vi "dg645-full-controll2_legacy.vi"(0 "Cluster":T1={"ch AB delay(ns)"=0.0, "ch AB width(ns)"=1020.0, "ch CD delay(ns) "=0.0, "ch CD width(ns) "=2000.0, "ch EF delay(ns) "=0.0, "ch EF width(ns) "=1000.0, "ch GH delay(ns) "=0.0, "ch GH width(ns) "=1000.0} {"ch GH width(ns)" format="%^#_6e"; "ch GH delay(ns)" format="%^#_6e"; "ch EF width(ns)" format="%^#_6e"; "ch EF delay(ns)" format="%^#_6e"; "ch CD width(ns)" format="%^#_6e"; "ch CD delay(ns)" format="%^#_6e"; "ch AB width(ns)" format="%^#_6e"; "ch AB delay(ns)" format="%^#_6e"}) -> ()   [LabVIEW 2018]
doc: "This VI is an example of how to use the DG535 subVIs programmatically .\nThe DG535 TRIGGER.VI sets the trigger mode , internal/burst trigger rate , burst count , burst period , external threshold voltage , external trigger slope and impedance of the DG535 .\nErrors are reported if the trigger rate is too high or if the burst period is out-of-range .\nThe DG535 DELAY.VI sets the delay time of channel i to t seconds relative to channel j . A \"Delay Linkage Error\" is caused by an attempt to totally disconnect a time reference from T0 . A \"Delay Range Error\" is reported when the total time delay for a channel exceeds 999.999999999995 seconds .\nDG535 SET OUTPUT.VI sets the mode , load , output polarity, amplitude and offset of the OUTPUT BNC selected while the DG535 READ OUTPUT.VI reads and displays these values ."
panel:
  in  "Tab Control":enum32{"delay ", "output level"}(tab)
  in  "Inhibit trigger?":bool
  out "chH delay from G":string="8,+0.000000000000\r\n"
  out "chF delay from E":string="6,+0.000100000000\r\n"
  out "chG delay from T0":string="0,+0.000000000000\r\n"
  out "chE delay from T0":string="0,+0.000000000000\r\n"
  out "chC delay from T0":string="0,+0.000000000000\r\n"
  out "chD delay from C":string="4,+0.000001000000\r\n"
  out "chB delay from A":string="2,+0.000000370000\r\n"
  out "chA delay from T0":string
  in  "save?":bool
  in  "ch GH width(ns)":dbl=1000.0 format="%^#_6e"
  in  "ch GH delay(ns)":dbl format="%^#_6e"
  in  "ch EF width(ns)":dbl=1000.0 format="%^#_6e"
  in  "ch EF delay(ns)":dbl format="%^#_6e"
  in  "ch CD width(ns)":dbl=2000.0 format="%^#_6e"
  in  "ch CD delay(ns)":dbl format="%^#_6e"
  in  "ch AB width(ns)":dbl=1020.0 format="%^#_6e"
  in  "ch AB delay(ns)":dbl format="%^#_6e"
  in  "GPIB Address":string="15"
  out "error out":errorcluster
  in  "error in":errorcluster
  # "ps"
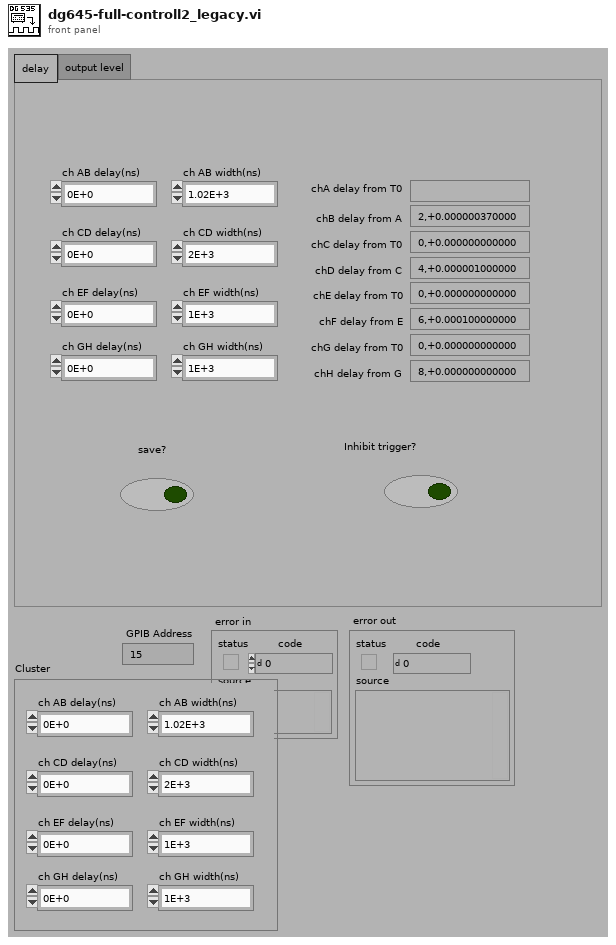
[diagram p1: front panel]
types:
  T1 = cluster{"ch AB delay(ns)":dbl, "ch AB width(ns)":dbl, "ch CD delay(ns) ":dbl, "ch CD width(ns) ":dbl, "ch EF delay(ns) ":dbl, "ch EF width(ns) ":dbl, "ch GH delay(ns) ":dbl, "ch GH width(ns) ":dbl}
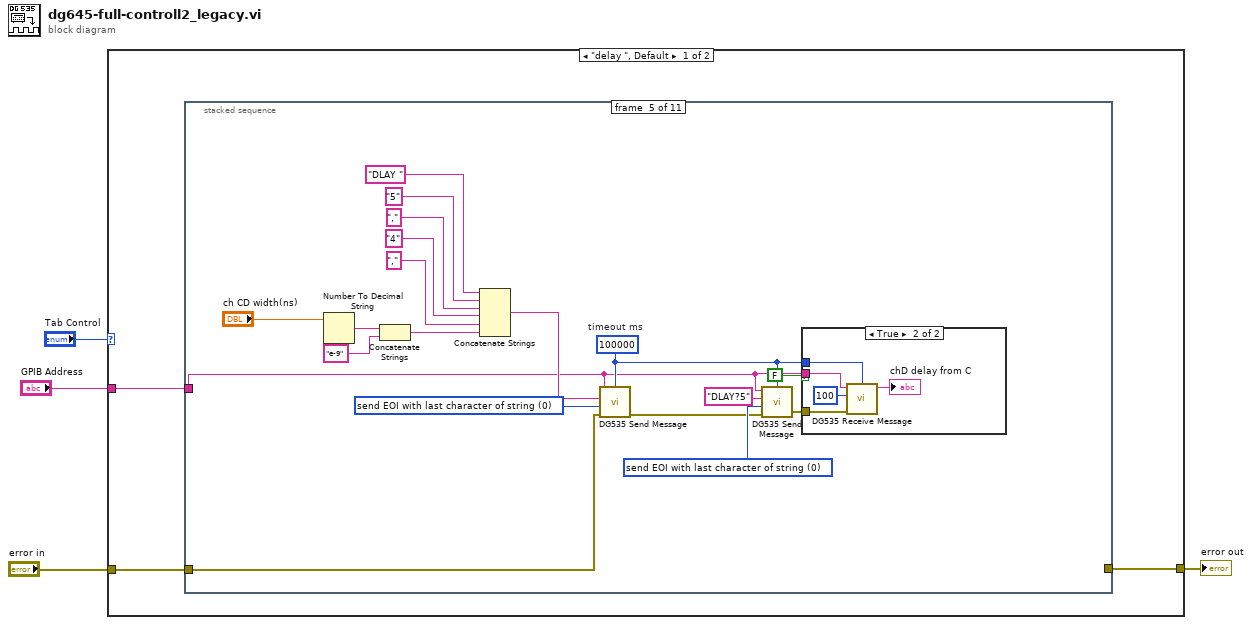
[diagram p0: block diagram]
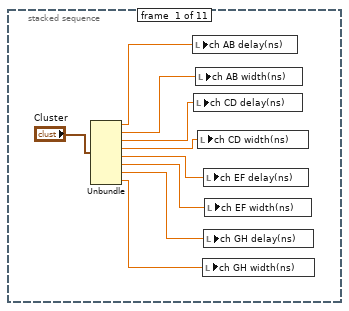
[diagram p2: hidden frame]
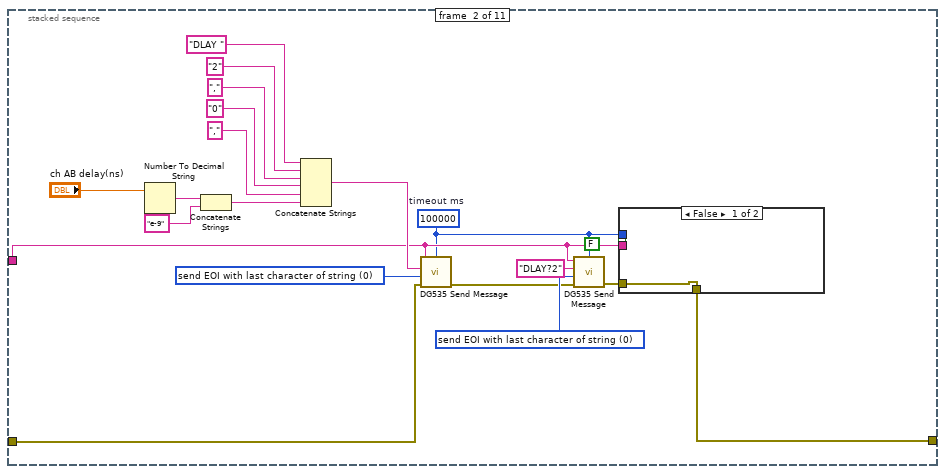
[diagram p3: hidden frame]
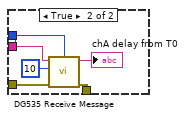
[diagram p4: hidden frame]
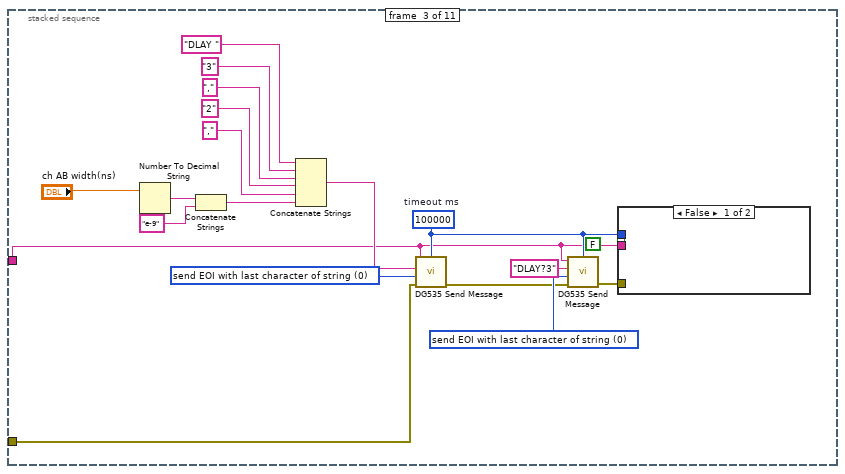
[diagram p5: hidden frame]
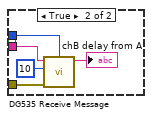
[diagram p6: hidden frame]
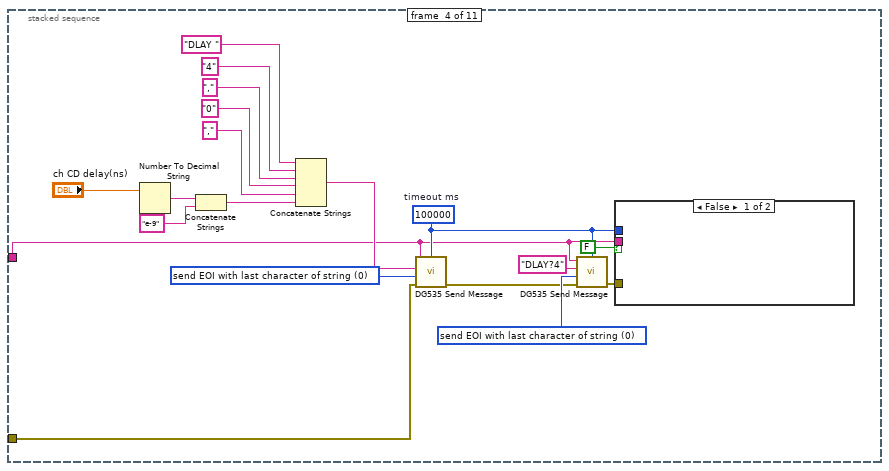
[diagram p7: hidden frame]
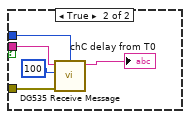
[diagram p8: hidden frame]
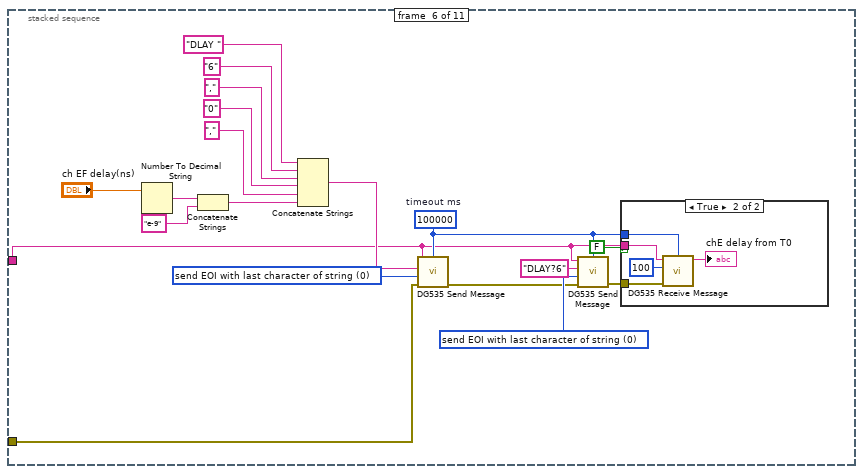
[diagram p10: hidden frame]
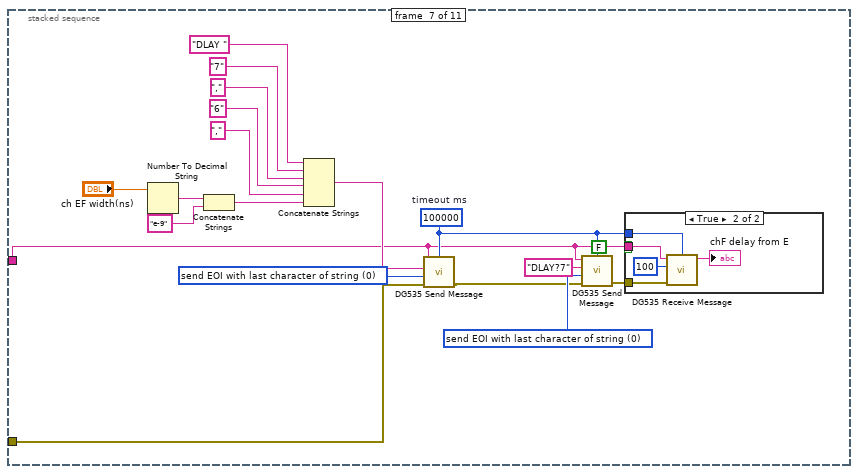
[diagram p12: hidden frame]
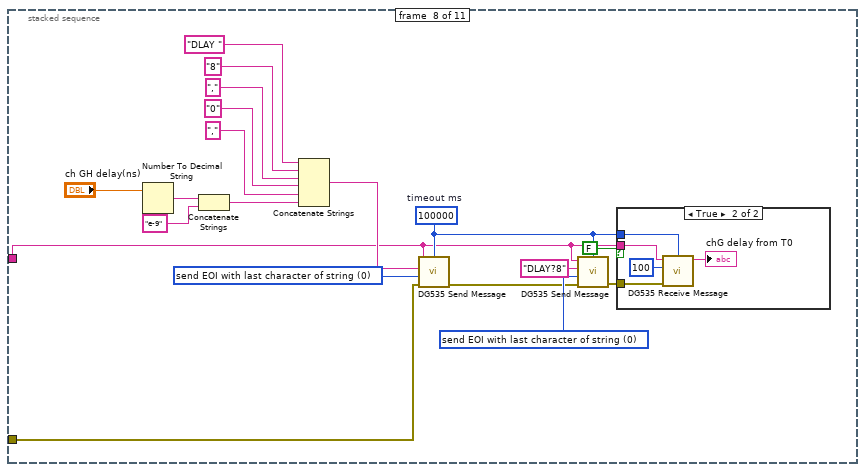
[diagram p14: hidden frame]
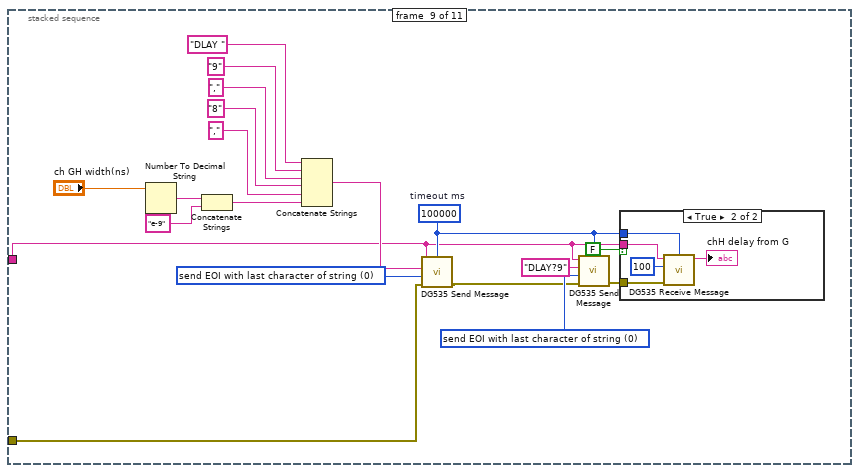
[diagram p16: hidden frame]
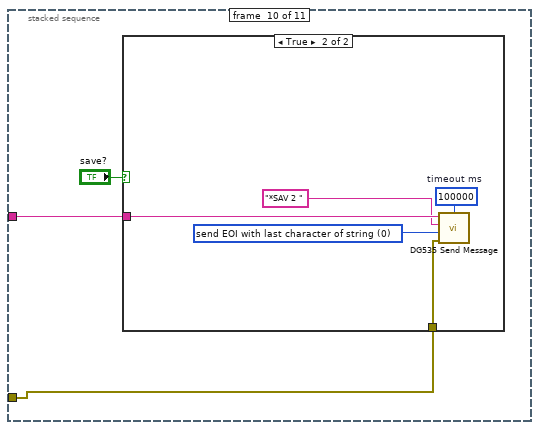
[diagram p18: hidden frame]
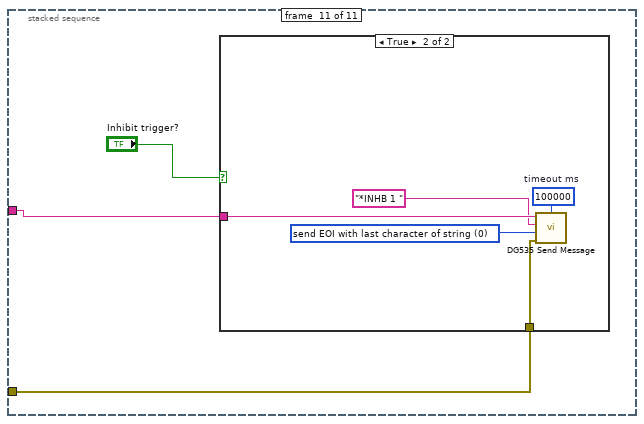
[diagram p20: hidden frame]
diagram:
  n1 = case shown="\"delay \", Default" "Tab Control" {
    tunnel: "error in" -> [w7 w233]
    tunnel: [w6 w233] -> w2
    tunnel: "GPIB Address" -> [w5 _]
    frame "delay ", Default {
      n2 = stacked-sequence {
        tunnel: w7 -> [_ w28 w53 w75 w100 w124 w147 w172 w196 w213 w220]
        tunnel: [_ w19 _ _ _ _ _ _ _ _ _] -> w6
        tunnel: w5 -> [_ w21 w46 w70 w93 w117 w141 w165 w189 w214 w221]
        frame #0 {
          n3 = Unbundle("Cluster") -> ("ch AB delay(ns)"=w15:dbl, "ch AB width(ns)"=w14:dbl, "ch CD delay(ns)"=w13:dbl, "ch CD width(ns)"=w12:dbl, "ch EF delay(ns)"=w11:dbl, "ch EF width(ns)"=w10:dbl, "ch GH delay(ns)"=w9:dbl, "ch GH width(ns)"=w8:dbl)
          n4 = local write "ch AB delay(ns)"(w15) -> ()
          n5 = local write "ch CD delay(ns)"(w13) -> ()
          n6 = local write "ch AB width(ns)"(w14) -> ()
          n7 = local write "ch CD width(ns)"(w12) -> ()
          n8 = local write "ch GH width(ns)"(w8) -> ()
          n9 = local write "ch EF delay(ns)"(w11) -> ()
          n10 = local write "ch GH delay(ns)"(w9) -> ()
          n11 = local write "ch EF width(ns)"(w10) -> ()
        }
        frame #1 {
          w25 = 0 items=["send EOI with last character of string", "append CR to string and send EOI with CR", "append LF to string and send EOI with LF", "append CR LF to string and send EOI with LF", "append CR to string but do not send EOI", "append LF to string but do not send EOI", "append CR LF to string but do not send EOI", "do not send EOI"] ("write mode (set END:0)")
          w17 = 0 items=["send EOI with last character of string", "append CR to string and send EOI with CR", "append LF to string and send EOI with LF", "append CR LF to string and send EOI with LF", "append CR to string but do not send EOI", "append LF to string but do not send EOI", "append CR LF to string but do not send EOI", "do not send EOI"] ("write mode (set END:0)")
          w20 = u32 100000  # timeout ms
          n12 = Number To Decimal String(number="ch AB delay(ns)") -> (decimal integer string=w29:string)  [unwired: 1 in]
          n13 = Concatenate Strings(w29, "e-9" ("string 2")) -> (w31:string)
          n14 = Concatenate Strings("DLAY " ("string"), "2" ("string"), "," ("string"), "0" ("string"), "," ("string"), w31) -> (w27:string)
          n15 = call "DG535 Send Message.vi"("timeout ms"=w20, "address string"=w21, "write buffer"=w27, "write mode (set END:0)"=w17, "error in"=w28) -> ("error out"=w24:errorcluster)  [unwired: 2 in, 2 out]
          n16 = call "DG535 Send Message.vi"("timeout ms"=w20, "address string"=w21, "write buffer"="DLAY?2", "write mode (set END:0)"=w25, "error in"=w24) -> ("error out"=w22:errorcluster)  [unwired: 2 in, 2 out]
          n17 = case shown="False" FALSE {
            tunnel: w22 -> [w37 w43]
            tunnel: w21 -> [_ w41]
            tunnel: w20 -> [_ w40]
            tunnel: [w37 w39] -> w19
            frame False {
            }
            frame True {
              n18 = call "DG535 Receive Message.vi"("timeout ms"=w40, "address string"=w41, "byte count"=10, "error in"=w43) -> ("read buffer"=→"chA delay from T0":string, "error out"=w39:errorcluster)  [unwired: 3 in, 1 out]
            }
          }
        }
        frame #2 {
          w48 = 0 items=["send EOI with last character of string", "append CR to string and send EOI with CR", "append LF to string and send EOI with LF", "append CR LF to string and send EOI with LF", "append CR to string but do not send EOI", "append LF to string but do not send EOI", "append CR LF to string but do not send EOI", "do not send EOI"] ("write mode (set END:0)")
          w61 = 0 items=["send EOI with last character of string", "append CR to string and send EOI with CR", "append LF to string and send EOI with LF", "append CR LF to string and send EOI with LF", "append CR to string but do not send EOI", "append LF to string but do not send EOI", "append CR LF to string but do not send EOI", "do not send EOI"] ("write mode (set END:0)")
          w47 = u32 100000  # timeout ms
          n19 = Number To Decimal String(number="ch AB width(ns)") -> (decimal integer string=w62:string)  [unwired: 1 in]
          n20 = Concatenate Strings(w62, "e-9" ("string 2")) -> (w59:string)
          n21 = Concatenate Strings("DLAY " ("string"), "3" ("string"), "," ("string"), "2" ("string"), "," ("string"), w59) -> (w52:string)
          n22 = call "DG535 Send Message.vi"("timeout ms"=w47, "address string"=w46, "write buffer"=w52, "write mode (set END:0)"=w61, "error in"=w53) -> ("error out"=w45:errorcluster)  [unwired: 2 in, 2 out]
          n23 = call "DG535 Send Message.vi"("timeout ms"=w47, "address string"=w46, "write buffer"="DLAY?3", "write mode (set END:0)"=w48, "error in"=w45) -> ("error out"=w50:errorcluster)  [unwired: 2 in, 2 out]
          n24 = case shown="False" FALSE {
            tunnel: w50 -> [_ w65]
            tunnel: w47 -> [_ w64]
            tunnel: w46 -> [_ w63]
            frame False {
            }
            frame True {
              n25 = call "DG535 Receive Message.vi"("timeout ms"=w64, "address string"=w63, "byte count"=10, "error in"=w65) -> ("read buffer"=→"chB delay from A":string)  [unwired: 3 in, 2 out]
            }
          }
        }
        frame #3 {
          w74 = 0 items=["send EOI with last character of string", "append CR to string and send EOI with CR", "append LF to string and send EOI with LF", "append CR LF to string and send EOI with LF", "append CR to string but do not send EOI", "append LF to string but do not send EOI", "append CR LF to string but do not send EOI", "do not send EOI"] ("write mode (set END:0)")
          w78 = 0 items=["send EOI with last character of string", "append CR to string and send EOI with CR", "append LF to string and send EOI with LF", "append CR LF to string and send EOI with LF", "append CR to string but do not send EOI", "append LF to string but do not send EOI", "append CR LF to string but do not send EOI", "do not send EOI"] ("write mode (set END:0)")
          w71 = u32 100000  # timeout ms
          n26 = Number To Decimal String(number="ch CD delay(ns)") -> (decimal integer string=w77:string)  [unwired: 1 in]
          n27 = Concatenate Strings(w77, "e-9" ("string 2")) -> (w80:string)
          n28 = Concatenate Strings("DLAY " ("string"), "4" ("string"), "," ("string"), "0" ("string"), "," ("string"), w80) -> (w86:string)
          n29 = call "DG535 Send Message.vi"("timeout ms"=w71, "address string"=w70, "write buffer"=w86, "write mode (set END:0)"=w78, "error in"=w75) -> ("error out"=w69:errorcluster)  [unwired: 2 in, 2 out]
          n30 = call "DG535 Send Message.vi"("timeout ms"=w71, "address string"=w70, "write buffer"="DLAY?4", "write mode (set END:0)"=w74, "error in"=w69) -> ("error out"=w72:errorcluster)  [unwired: 2 in, 2 out]
          n31 = case shown="False" FALSE {
            tunnel: w72 -> [_ w91]
            tunnel: w71 -> [_ w88]
            tunnel: w70 -> [_ w87]
            frame False {
            }
            frame True {
              n32 = call "DG535 Receive Message.vi"("timeout ms"=w88, "address string"=w87, "byte count"=100, "error in"=w91) -> ("read buffer"=→"chC delay from T0":string)  [unwired: 3 in, 2 out]
            }
          }
        }
        frame #4 {
          w98 = 0 items=["send EOI with last character of string", "append CR to string and send EOI with CR", "append LF to string and send EOI with LF", "append CR LF to string and send EOI with LF", "append CR to string but do not send EOI", "append LF to string but do not send EOI", "append CR LF to string but do not send EOI", "do not send EOI"] ("write mode (set END:0)")
          w102 = 0 items=["send EOI with last character of string", "append CR to string and send EOI with CR", "append LF to string and send EOI with LF", "append CR LF to string and send EOI with LF", "append CR to string but do not send EOI", "append LF to string but do not send EOI", "append CR LF to string but do not send EOI", "do not send EOI"] ("write mode (set END:0)")
          w95 = u32 100000  # timeout ms
          n33 = Number To Decimal String(number="ch CD width(ns)") -> (decimal integer string=w101:string)  [unwired: 1 in]
          n34 = Concatenate Strings(w101, "e-9" ("string 2")) -> (w104:string)
          n35 = Concatenate Strings("DLAY " ("string"), "5" ("string"), "," ("string"), "4" ("string"), "," ("string"), w104) -> (w110:string)
          n36 = call "DG535 Send Message.vi"("timeout ms"=w95, "address string"=w93, "write buffer"=w110, "write mode (set END:0)"=w102, "error in"=w100) -> ("error out"=w94:errorcluster)  [unwired: 2 in, 2 out]
          n37 = call "DG535 Send Message.vi"("timeout ms"=w95, "address string"=w93, "write buffer"="DLAY?5", "write mode (set END:0)"=w98, "error in"=w94) -> ("error out"=w96:errorcluster)  [unwired: 2 in, 2 out]
          n38 = case shown="True" FALSE {
            tunnel: w96 -> [_ w115]
            tunnel: w95 -> [_ w112]
            tunnel: w93 -> [_ w111]
            frame False {
            }
            frame True {
              n39 = call "DG535 Receive Message.vi"("timeout ms"=w112, "address string"=w111, "byte count"=100, "error in"=w115) -> ("read buffer"=→"chD delay from C":string)  [unwired: 3 in, 2 out]
            }
          }
        }
        frame #5 {
          w122 = 0 items=["send EOI with last character of string", "append CR to string and send EOI with CR", "append LF to string and send EOI with LF", "append CR LF to string and send EOI with LF", "append CR to string but do not send EOI", "append LF to string but do not send EOI", "append CR LF to string but do not send EOI", "do not send EOI"] ("write mode (set END:0)")
          w126 = 0 items=["send EOI with last character of string", "append CR to string and send EOI with CR", "append LF to string and send EOI with LF", "append CR LF to string and send EOI with LF", "append CR to string but do not send EOI", "append LF to string but do not send EOI", "append CR LF to string but do not send EOI", "do not send EOI"] ("write mode (set END:0)")
          w118 = u32 100000  # timeout ms
          n40 = Number To Decimal String(number="ch EF delay(ns)") -> (decimal integer string=w125:string)  [unwired: 1 in]
          n41 = Concatenate Strings(w125, "e-9" ("string 2")) -> (w128:string)
          n42 = Concatenate Strings("DLAY " ("string"), "6" ("string"), "," ("string"), "0" ("string"), "," ("string"), w128) -> (w134:string)
          n43 = call "DG535 Send Message.vi"("timeout ms"=w118, "address string"=w117, "write buffer"=w134, "write mode (set END:0)"=w126, "error in"=w124) -> ("error out"=w119:errorcluster)  [unwired: 2 in, 2 out]
          n44 = call "DG535 Send Message.vi"("timeout ms"=w118, "address string"=w117, "write buffer"="DLAY?6", "write mode (set END:0)"=w122, "error in"=w119) -> ("error out"=w120:errorcluster)  [unwired: 2 in, 2 out]
          n45 = case shown="True" FALSE {
            tunnel: w120 -> [_ w139]
            tunnel: w118 -> [_ w136]
            tunnel: w117 -> [_ w135]
            frame False {
            }
            frame True {
              n46 = call "DG535 Receive Message.vi"("timeout ms"=w136, "address string"=w135, "byte count"=100, "error in"=w139) -> ("read buffer"=→"chE delay from T0":string)  [unwired: 3 in, 2 out]
            }
          }
        }
        frame #6 {
          w146 = 0 items=["send EOI with last character of string", "append CR to string and send EOI with CR", "append LF to string and send EOI with LF", "append CR LF to string and send EOI with LF", "append CR to string but do not send EOI", "append LF to string but do not send EOI", "append CR LF to string but do not send EOI", "do not send EOI"] ("write mode (set END:0)")
          w150 = 0 items=["send EOI with last character of string", "append CR to string and send EOI with CR", "append LF to string and send EOI with LF", "append CR LF to string and send EOI with LF", "append CR to string but do not send EOI", "append LF to string but do not send EOI", "append CR LF to string but do not send EOI", "do not send EOI"] ("write mode (set END:0)")
          w142 = u32 100000  # timeout ms
          n47 = Number To Decimal String(number="ch EF width(ns)") -> (decimal integer string=w149:string)  [unwired: 1 in]
          n48 = Concatenate Strings(w149, "e-9" ("string 2")) -> (w152:string)
          n49 = Concatenate Strings("DLAY " ("string"), "7" ("string"), "," ("string"), "6" ("string"), "," ("string"), w152) -> (w158:string)
          n50 = call "DG535 Send Message.vi"("timeout ms"=w142, "address string"=w141, "write buffer"=w158, "write mode (set END:0)"=w150, "error in"=w147) -> ("error out"=w143:errorcluster)  [unwired: 2 in, 2 out]
          n51 = call "DG535 Send Message.vi"("timeout ms"=w142, "address string"=w141, "write buffer"="DLAY?7", "write mode (set END:0)"=w146, "error in"=w143) -> ("error out"=w144:errorcluster)  [unwired: 2 in, 2 out]
          n52 = case shown="True" FALSE {
            tunnel: w144 -> [_ w163]
            tunnel: w142 -> [_ w160]
            tunnel: w141 -> [_ w159]
            frame False {
            }
            frame True {
              n53 = call "DG535 Receive Message.vi"("timeout ms"=w160, "address string"=w159, "byte count"=100, "error in"=w163) -> ("read buffer"=→"chF delay from E":string)  [unwired: 3 in, 2 out]
            }
          }
        }
        frame #7 {
          w170 = 0 items=["send EOI with last character of string", "append CR to string and send EOI with CR", "append LF to string and send EOI with LF", "append CR LF to string and send EOI with LF", "append CR to string but do not send EOI", "append LF to string but do not send EOI", "append CR LF to string but do not send EOI", "do not send EOI"] ("write mode (set END:0)")
          w174 = 0 items=["send EOI with last character of string", "append CR to string and send EOI with CR", "append LF to string and send EOI with LF", "append CR LF to string and send EOI with LF", "append CR to string but do not send EOI", "append LF to string but do not send EOI", "append CR LF to string but do not send EOI", "do not send EOI"] ("write mode (set END:0)")
          w167 = u32 100000  # timeout ms
          n54 = Number To Decimal String(number="ch GH delay(ns)") -> (decimal integer string=w173:string)  [unwired: 1 in]
          n55 = Concatenate Strings(w173, "e-9" ("string 2")) -> (w176:string)
          n56 = Concatenate Strings("DLAY " ("string"), "8" ("string"), "," ("string"), "0" ("string"), "," ("string"), w176) -> (w182:string)
          n57 = call "DG535 Send Message.vi"("timeout ms"=w167, "address string"=w165, "write buffer"=w182, "write mode (set END:0)"=w174, "error in"=w172) -> ("error out"=w166:errorcluster)  [unwired: 2 in, 2 out]
          n58 = call "DG535 Send Message.vi"("timeout ms"=w167, "address string"=w165, "write buffer"="DLAY?8", "write mode (set END:0)"=w170, "error in"=w166) -> ("error out"=w168:errorcluster)  [unwired: 2 in, 2 out]
          n59 = case shown="True" FALSE {
            tunnel: w168 -> [_ w187]
            tunnel: w167 -> [_ w184]
            tunnel: w165 -> [_ w183]
            frame False {
            }
            frame True {
              n60 = call "DG535 Receive Message.vi"("timeout ms"=w184, "address string"=w183, "byte count"=100, "error in"=w187) -> ("read buffer"=→"chG delay from T0":string)  [unwired: 3 in, 2 out]
            }
          }
        }
        frame #8 {
          w194 = 0 items=["send EOI with last character of string", "append CR to string and send EOI with CR", "append LF to string and send EOI with LF", "append CR LF to string and send EOI with LF", "append CR to string but do not send EOI", "append LF to string but do not send EOI", "append CR LF to string but do not send EOI", "do not send EOI"] ("write mode (set END:0)")
          w198 = 0 items=["send EOI with last character of string", "append CR to string and send EOI with CR", "append LF to string and send EOI with LF", "append CR LF to string and send EOI with LF", "append CR to string but do not send EOI", "append LF to string but do not send EOI", "append CR LF to string but do not send EOI", "do not send EOI"] ("write mode (set END:0)")
          w190 = u32 100000  # timeout ms
          n61 = Number To Decimal String(number="ch GH width(ns)") -> (decimal integer string=w197:string)  [unwired: 1 in]
          n62 = Concatenate Strings(w197, "e-9" ("string 2")) -> (w200:string)
          n63 = Concatenate Strings("DLAY " ("string"), "9" ("string"), "," ("string"), "8" ("string"), "," ("string"), w200) -> (w206:string)
          n64 = call "DG535 Send Message.vi"("timeout ms"=w190, "address string"=w189, "write buffer"=w206, "write mode (set END:0)"=w198, "error in"=w196) -> ("error out"=w191:errorcluster)  [unwired: 2 in, 2 out]
          n65 = call "DG535 Send Message.vi"("timeout ms"=w190, "address string"=w189, "write buffer"="DLAY?9", "write mode (set END:0)"=w194, "error in"=w191) -> ("error out"=w192:errorcluster)  [unwired: 2 in, 2 out]
          n66 = case shown="True" FALSE {
            tunnel: w192 -> [_ w211]
            tunnel: w190 -> [_ w208]
            tunnel: w189 -> [_ w207]
            frame False {
            }
            frame True {
              n67 = call "DG535 Receive Message.vi"("timeout ms"=w208, "address string"=w207, "byte count"=100, "error in"=w211) -> ("read buffer"=→"chH delay from G":string)  [unwired: 3 in, 2 out]
            }
          }
        }
        frame #9 {
          n68 = case shown="True" "save?" {
            tunnel: w214 -> [_ w217]
            tunnel: w213 -> [_ w215]
            frame False {
            }
            frame True {
              w219 = 0 items=["send EOI with last character of string", "append CR to string and send EOI with CR", "append LF to string and send EOI with LF", "append CR LF to string and send EOI with LF", "append CR to string but do not send EOI", "append LF to string but do not send EOI", "append CR LF to string but do not send EOI", "do not send EOI"] ("write mode (set END:0)")
              w218 = u32 100000  # timeout ms
              n69 = call "DG535 Send Message.vi"("timeout ms"=w218, "address string"=w217, "write buffer"="*SAV 2 " ("string"), "write mode (set END:0)"=w219, "error in"=w215) -> ()  [unwired: 2 in, 3 out]
            }
          }
        }
        frame #10 {
          n70 = case shown="True" "Inhibit trigger?" {
            tunnel: w221 -> [w224 w230]
            tunnel: w220 -> [w223 w228]
            frame False {
              w227 = 0 items=["send EOI with last character of string", "append CR to string and send EOI with CR", "append LF to string and send EOI with LF", "append CR LF to string and send EOI with LF", "append CR to string but do not send EOI", "append LF to string but do not send EOI", "append CR LF to string but do not send EOI", "do not send EOI"] ("write mode (set END:0)")
              w226 = u32 100000  # timeout ms
              n71 = call "DG535 Send Message.vi"("timeout ms"=w226, "address string"=w224, "write buffer"="*INHB 0 " ("string"), "write mode (set END:0)"=w227, "error in"=w223) -> ()  [unwired: 2 in, 3 out]
            }
            frame True {
              w232 = 0 items=["send EOI with last character of string", "append CR to string and send EOI with CR", "append LF to string and send EOI with LF", "append CR LF to string and send EOI with LF", "append CR to string but do not send EOI", "append LF to string but do not send EOI", "append CR LF to string but do not send EOI", "do not send EOI"] ("write mode (set END:0)")
              w231 = u32 100000  # timeout ms
              n72 = call "DG535 Send Message.vi"("timeout ms"=w231, "address string"=w230, "write buffer"="*INHB 1 " ("string"), "write mode (set END:0)"=w232, "error in"=w228) -> ()  [unwired: 2 in, 3 out]
            }
          }
        }
      }
    }
    frame "output level" {
    }
  }
  "error out" <- w2
